vi "SRV_Write_Comm_sub.vi"(8 "error in (no error)":errorcluster, 10 "Command Sent":string, 11 "SRV In":refnum<k5>) -> (0 "error out":errorcluster, 2 "Command Sent dup":string, 3 "SRV Out":refnum<k5>)   [LabVIEW 2009]
doc: "Writes a string to the SRV.\n\n\nWritten for Benilde St. Margaret's School - Tim Jump\nBy Doug Schmertman - Logic PD\nCopyright 2012"
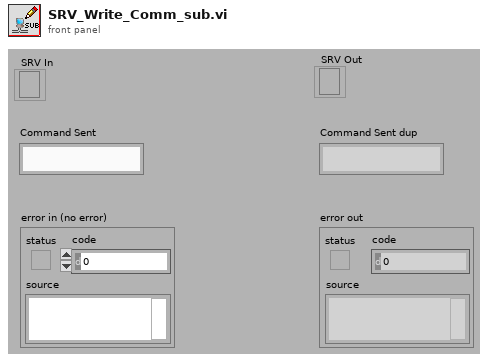
[diagram p1: front panel]
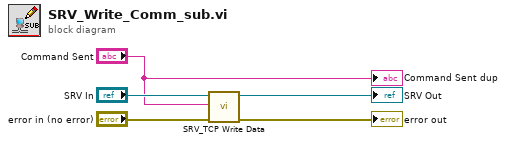
[diagram p0: block diagram]
diagram:
  n1 = call "SRV_TCP Write Data.vi"("error in"="error in (no error)", "data in"="Command Sent", "connection ID"="SRV In") -> ("error out"=→"error out":errorcluster, "connection ID out"=→"SRV Out":refnum<k5>)  [unwired: 6 in, 1 out]
  "Command Sent dup" <- "Command Sent"
